vi "GetMetadataCount.vi"(7 "DLL path":path, 8 "error in (no error)":errorcluster, 11 "session id in":i32) -> (0 "error out":errorcluster, 2 "MetadataCount":i32, 3 "session id out":i32)   [LabVIEW 2017, in "ONNX Class Library.lvlib"]
doc: "/**\n * @brief Получить количество метаданных модели\n * \n * ONNX модели могут содержать метаданные: версию, имя автора, описание и т.д.\n * \n * @param sessionId [IN] ID сессии\n * \n * @return int32: Количество пар ключ-значение\n * @return int32: 0 если сессия не найдена или метаданных нет\n */\nint GetMetadataCount(int sessionId);"
uses:
  ONNX Class Library.lvlib
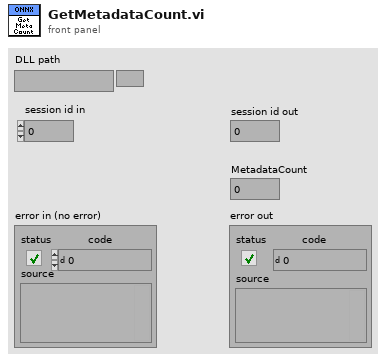
[diagram p1: front panel]
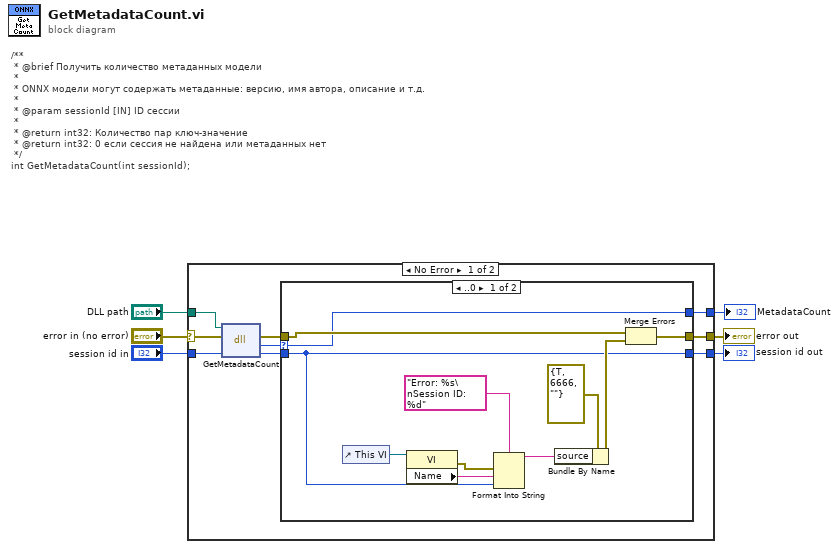
[diagram p0: block diagram]
diagram:
  # "/**\n * @brief Получить количество метаданных модели\n * \n * ONNX модели могут содержать метаданные: версию, имя автора, описание и т.д.\n * \n * @param sessionId [IN] ID сессии\n * \n * @return int32: Количество пар ключ-значение\n * @return int32: 0 если сессия не найдена или метаданных нет\n */\nint GetMetadataCount(int sessionId);"
  n1 = case shown="No Error" "error in (no error)" {
    selector: "error in (no error)" -> [w8 w31]
    tunnel: "session id in" -> [w15 w30]
    tunnel: [w11 w31] -> w5
    tunnel: [w10 _] -> w4
    tunnel: [w9 w30] -> w3
    tunnel: "DLL path" -> [w7 _]
    frame No Error {
      n2 = dll-call lib="home/ivan/LabVIEWData/ONNX/Test/libonnx_wrapper/unix64/libonnx_wrapper.so" fn="GetMetadataCount"(path in=w7, error in=w8, "sessionId"=w15) -> (error out=w14:errorcluster, "MetadataCount"=w13:i32, "sessionId"=w12:i32)  [unwired: 1 in, 1 out]
      n3 = case shown="..0" w13 {
        selector: w13 -> [w16 w27]
        tunnel: w14 -> [w17 w29]
        tunnel: [w18 w29] -> w11
        tunnel: w12 -> [w19 w28]
        tunnel: [w19 w28] -> w9
        tunnel: [w16 w27] -> w10
        frame ..0 {
          n4 = control-ref of="This VI"() -> (w23:refnum<vi>)
          n5 = property class="VI"(reference=w23) -> (error out=w20:errorcluster, "Name"=w22:string)  [unwired: 1 in, 1 out]
          n6 = Format Into String(format string="Error: %s\nSession ID: %d", error in=w20, w22, w19) -> (resulting string=w24:string)  [unwired: 1 in, 1 out]
          n7 = Bundle By Name(cluster=errorcluster {"status"=TRUE, "code"=6666, "source"=""} ("error out"), "source"=w24) -> (w25:errorcluster)
          n8 = Merge Errors(w17, w25) -> (w18:errorcluster)
        }
        frame 1.. {
        }
      }
    }
    frame Error {
    }
  }
  "error out" <- w5
  "session id out" <- w3
  "MetadataCount" <- w4
